vi "SearchTarget.vi"(8 "error in (no error)":errorcluster, 10 "Game":refnum<class "Game.lvclass">, 11 "object in":refnum<class "Zone.lvclass">) -> (0 "error out":errorcluster, 3 "object out":refnum<class "Zone.lvclass">)   [LabVIEW 2023, in "Zone.lvclass"]
uses:
  Zone.lvclass
  Game_class/Game.lvclass
  Game_class/Game.lvclass/Game.ctl
  Parameters_class/Parameters.lvclass/Parameters.ctl
  Game_class/Read Parameters.lvclass.vi
  Parameters_class/Read AttakingOurselves.vi
  Game_class/Read FieldRef.vi
  Field_class/Field.lvclass
  Parameters_class/Parameters.lvclass
  Utilities_class/Utilities.lvclass
panel:
  in  "targetPosition":dbl[](array[numeric])
  in  "Divisor":dbl=2.0 format="%#_13g"
  in  "NumberOfSamples":i32=20
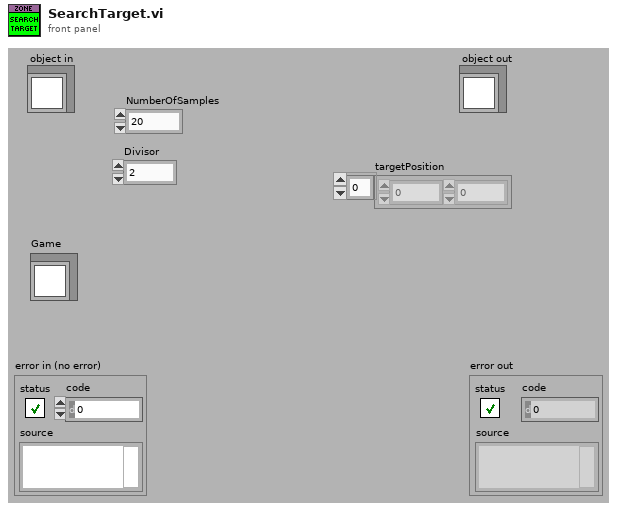
[diagram p1: front panel]
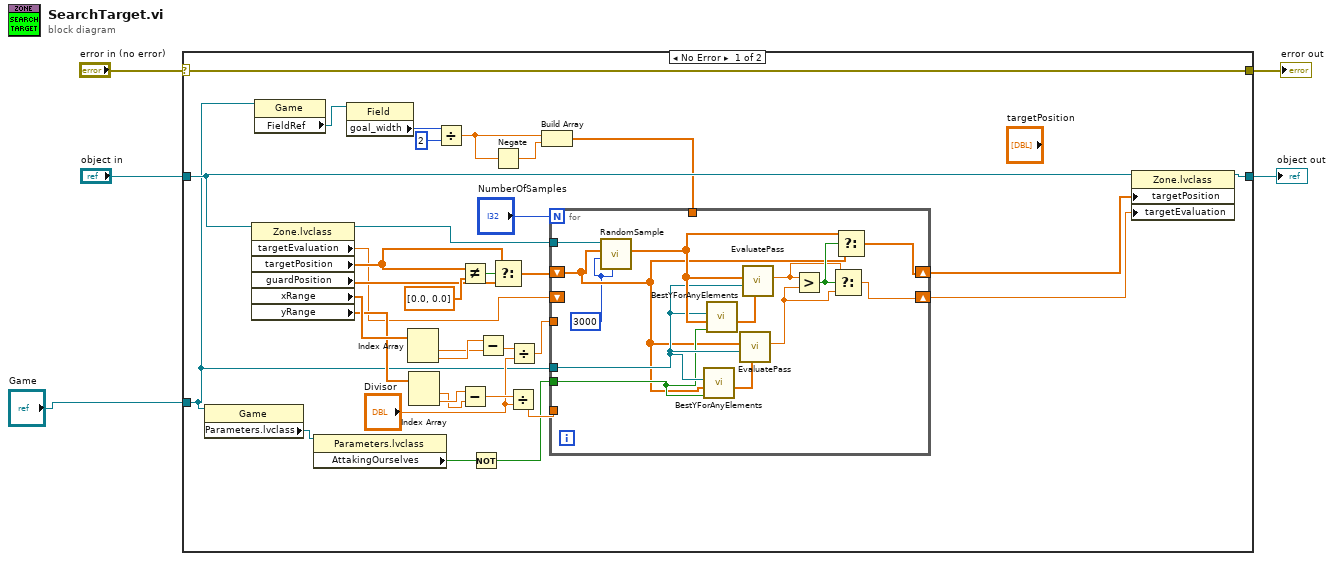
[diagram p0: block diagram]
diagram:
  n1 = case shown="No Error" "error in (no error)" {
    selector: "error in (no error)" -> [w39 w54]
    tunnel: [w39 w54] -> w4
    tunnel: [w37 w53] -> w2
    tunnel: "object in" -> [w38 w53]
    tunnel: "Game" -> [w12 _]
    frame No Error {
      n2 = property class="Game"(reference=w12) -> ("Parameters.lvclass"=w11:refnum<class "Parameters.lvclass">)  [unwired: 1 in, 2 out]
      n3 = property class="Zone.lvclass"(reference=w38) -> (reference out=w35:refnum<class "Zone.lvclass">, "targetEvaluation"=w19:dbl, "targetPosition"=w31:dbl[], "guardPosition"=w32:dbl[], "xRange"=w30:dbl[], "yRange"=w29:dbl[])  [unwired: 1 in, 1 out]
      n4 = property class="Game"(reference=w12) -> ("FieldRef"=w18:refnum<class "Field.lvclass">)  [unwired: 1 in, 2 out]
      n5 = property class="Parameters.lvclass"(reference=w11) -> ("AttakingOurselves"=w10:bool)  [unwired: 1 in, 2 out]
      n6 = property class="Field"(reference=w18) -> ("goal_width"=w17:i32)  [unwired: 1 in, 2 out]
      n7 = Index Array(array=w30) -> (element #1=w27:dbl, element #2=w28:dbl)  [unwired: 2 in]
      n8 = Index Array(array=w29) -> (element #1=w25:dbl, element #2=w26:dbl)  [unwired: 2 in]
      n9 = Divide(x=w17, y=2) -> (x/y=w14:dbl)
      n10 = Not Equal?(x=w31, y=dbl[] [0.0, 0.0]) -> (x != y?=w33:bool)
      n11 = Subtract(x=w26, y=w25) -> (x-y=w24:dbl)
      n12 = Not(x=w10) -> (.not. x?=w9:bool)
      n13 = Subtract(x=w28, y=w27) -> (x-y=w8:dbl)
      n14 = Negate(x=w14) -> (-x=w15:dbl)
      n15 = Select(t=w31, s=w33, f=w32) -> (s? t:f=w20:dbl[])
      n16 = Divide(x=w24, y="Divisor") -> (x/y=w21:dbl)
      n17 = Divide(x=w8, y="Divisor") -> (x/y=w22:dbl)
      n18 = Build Array(w14, w15) -> (w13:dbl[])
      n19 = for {
        N: "NumberOfSamples" -> [_]
        tunnel: w35 -> [w52]
        shift-right: [w49] -> w7
        shift-left: w20 -> [w41]
        tunnel: w12 -> [w43]
        tunnel: w22 -> [_]
        tunnel: w21 -> [_]
        shift-right: [w51] -> w6
        shift-left: w19 -> [_]
        tunnel: w13 -> [_]
        tunnel: w9 -> [w42]
        w40 = 3000
        n20 = call "RandomSample.vi"("widthStep"=w40, "lenghtStep"=w40, "basePoint"=w41, "object in"=w52) -> ("randomPoint"=w46:dbl[])  [unwired: 5 in, 2 out]
        n21 = call "BestYForAnyElements.vi"("inimigos"=w42, "Position to be analyzed"=w41, "Game"=w43) -> ("Gap Coord"=w45:dbl[])  [unwired: 5 in, 3 out]
        n22 = call "BestYForAnyElements.vi"("inimigos"=w42, "Position to be analyzed"=w46, "Game"=w43) -> ("Gap Coord"=w47:dbl[])  [unwired: 5 in, 3 out]
        n23 = call "EvaluatePass.vi"("Gap Coord"=w45, "Game"=w43, "Point"=w41) -> ("evaluation"=w44:dbl)  [unwired: 6 in, 2 out]
        n24 = call "EvaluatePass.vi"("Gap Coord"=w47, "Game"=w43, "Point"=w46) -> ("evaluation"=w48:dbl)  [unwired: 6 in, 2 out]
        n25 = Greater?(x=w48, y=w44) -> (0:w50:bool)
        n26 = Select(t=w48, s=w50, f=w44) -> (s? t:f=w51:dbl)
        n27 = Select(t=w46, s=w50, f=w41) -> (s? t:f=w49:dbl[])
      }
      n28 = property class="Zone.lvclass"(reference=w38, "targetPosition"=w7, "targetEvaluation"=w6) -> (reference out=w37:refnum<class "Zone.lvclass">)  [unwired: 1 in, 1 out]
    }
    frame Error {
    }
  }
  "error out" <- w4
  "object out" <- w2
